vi "PID++ Change Detect.vi"(8 "P":dbl, 9 "I":dbl, 10 "D":dbl, 11 "FF":dbl) -> (2 "Changed?":bool)   [LabVIEW 2015]
uses:
  Common Code/Change Detect Double.vi
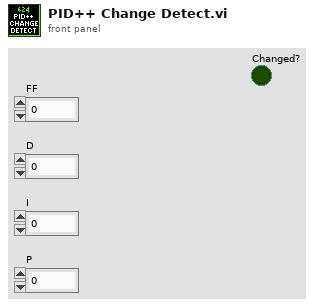
[diagram p1: front panel]
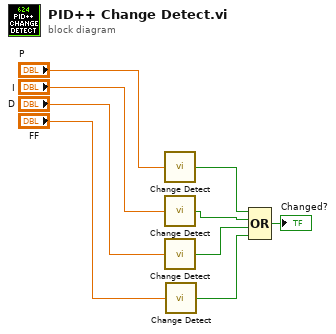
[diagram p0: block diagram]
diagram:
  n1 = call-poly "Change Detect.vi"("In"="P") -> ("Changed?"=w6:bool)
  n2 = call-poly "Change Detect.vi"("In"="I") -> ("Changed?"=w7:bool)
  n3 = call-poly "Change Detect.vi"("In"="D") -> ("Changed?"=w8:bool)
  n4 = call-poly "Change Detect.vi"("In"="FF") -> ("Changed?"=w9:bool)
  n5 = Compound Arithmetic op=OR(w6, w7, w8, w9) -> (→"Changed?":bool)
